vi "Main.vi"(10 "Acq Panel":refnum<vi>, 11 "Module Admin":refnum<class "Delacor_lib_QMH_Module Admin.lvclass">) -> ()   [LabVIEW 2019, in "Adquirir.lvlib"]
doc: "This template is based off of the Queued Message Handler design pattern and the Queued Message Handler project template that ships with LabVIEW.\n\nThe main difference is that the queue is private to this module and communication between modules is performed via Broadcast and Request events.\n\nRequest events are wrapped in public API methods and are handled in the Event Handling Loop (EHL) of this VI. Any module can register for Broadcast events sent by this module. The EHL generates messages based on user interface actions.\n\nThe Message Handling Loop (MHL) processes messages generated by the EHL, or by other messages. The messages are string values, so new messages can be added easily to the Message Cases case structure in the MHL. Each message cluster can also provide an optional value for Message Data, which is a variant that can be converted to whatever message-specific data is required.\n_____\nBased on Delacor QMH Project Template 5.0.0.82."
uses:
  Adquirir.lvlib
  <vilib>/Delacor/Delacor QMH/Libraries/Module Admin_class/Delacor_lib_QMH_Module Admin.lvclass
  Module Data--cluster.ctl
  Stop helper loop Argument--cluster.ctl
  <vilib>/Delacor/Delacor QMH/Libraries/Message Queue_class/Delacor_lib_QMH_Message Queue.lvclass/Delacor_lib_QMH_Message Queue.ctl
  Stop Argument--cluster.ctl
  <vilib>/Delacor/Delacor QMH/Libraries/Module Admin_class/Delacor_lib_QMH_Module Admin.lvclass/Delacor_lib_QMH_Module Admin.ctl
  <vilib>/Utility/miscctls.llb/LVPointTypeDef.ctl
  <vilib>/Delacor/Delacor QMH/Libraries/Message Queue_class/Delacor_lib_QMH_Enqueue Message (Single).vi
  <vilib>/Delacor/Delacor QMH/Libraries/Module Admin_class/Delacor_lib_QMH_Get External Launch.vi
  <vilib>/Utility/error.llb/Error Cluster From Error Code.vi
  <vilib>/ErrorRing/Error Ring.xnode
  <vilib>/Delacor/Delacor QMH/Libraries/Message Queue_class/Delacor_lib_QMH_Message Queue.lvclass
panel:
  out "Time Stamp":timestamp
  in  "Simulate MHL Error":bool
  in  "Simulate EHL Error":bool
  out "error out":errorcluster
  out "Status":string
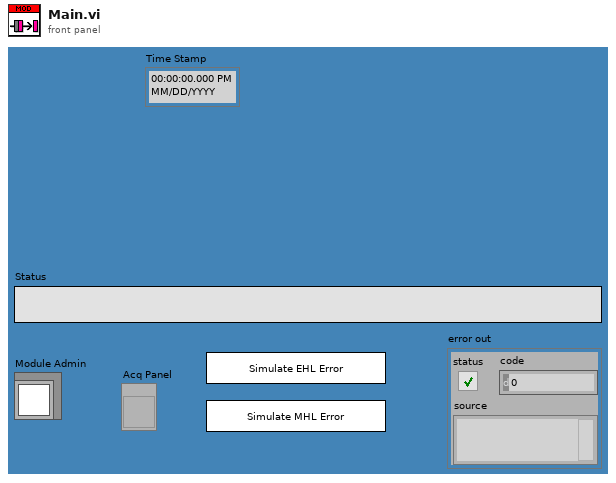
[diagram p1: front panel]
types:
  T1 = typedef "Adquirir.lvlib/Request Events--cluster.ctl" = cluster{"Stop Module":refnum<user-event>, "Show Panel":refnum<user-event>, "Hide Panel":refnum<user-event>, "Get Module Execution Status":refnum<user-event>, "Show Diagram":refnum<user-event>, "Start Helper Loop":refnum<user-event>, "Stop helper loop":refnum<user-event>}
  T2 = typedef "Adquirir.lvlib/Module Data--cluster.ctl" = cluster{"Status":string}
  T3 = typedef "Adquirir.lvlib/Stop helper loop Argument--cluster.ctl" = cluster{"Boolean":bool}
  T4 = enum32{"invalid lock state", "Not Locked", "Locked (No Password)", "Password-protected"}
  T5 = typedef "Adquirir.lvlib/Stop Argument--cluster.ctl" = cluster{"Origin":string, "Exit via Stop Module Req?":bool, "Wait for Module to stop?":bool}
  T6 = typedef "LVPointTypeDef.ctl" = cluster{"Horizontal":i16, "Vertical":i16}
  T7 = enum32{"Invalid", "Standard", "Closed", "Hidden", "Minimized", "Maximized"}
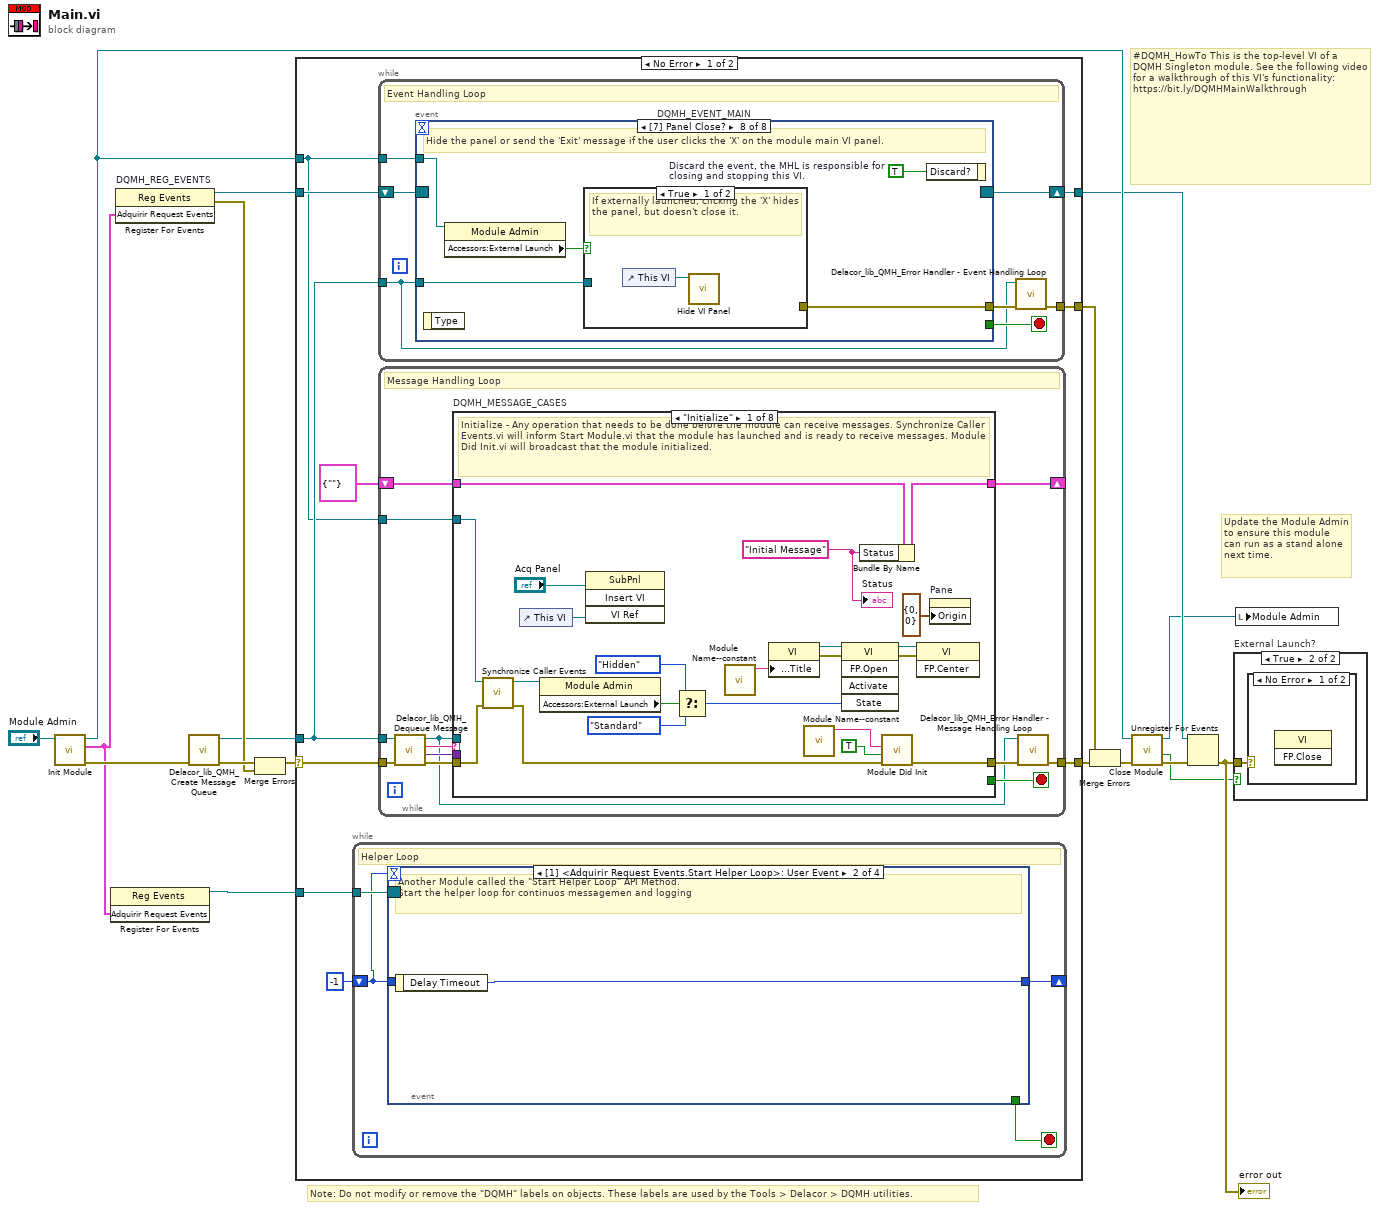
[diagram p0: block diagram]
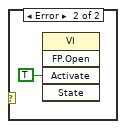
[diagram p3: hidden frame]
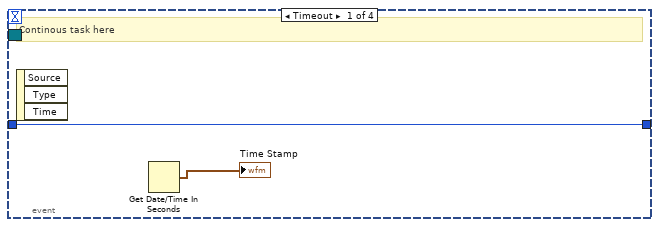
[diagram p4: hidden frame]
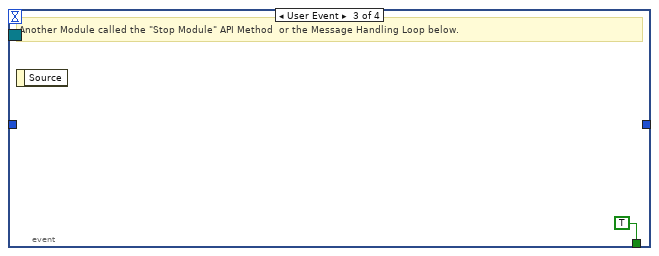
[diagram p5: hidden frame]
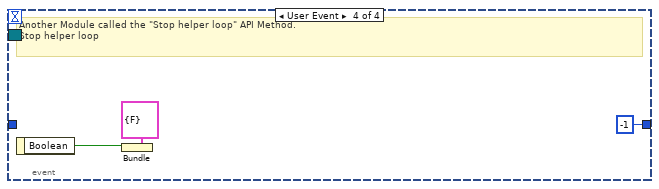
[diagram p6: hidden frame]
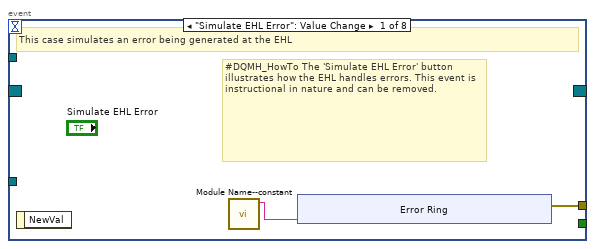
[diagram p7: hidden frame]
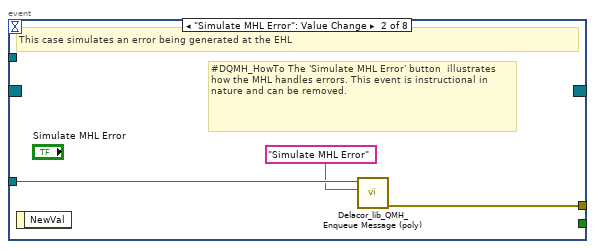
[diagram p8: hidden frame]
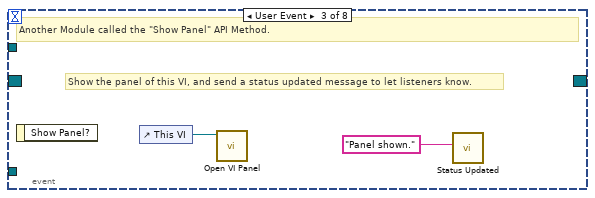
[diagram p9: hidden frame]
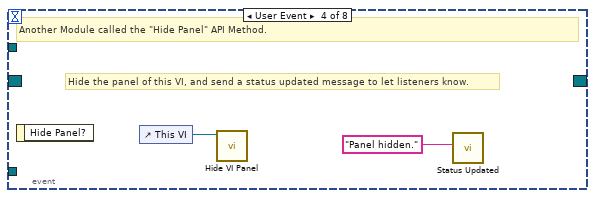
[diagram p10: hidden frame]
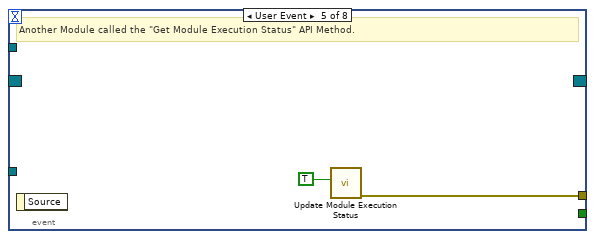
[diagram p11: hidden frame]
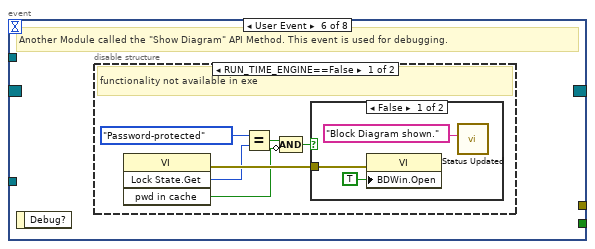
[diagram p12: hidden frame]
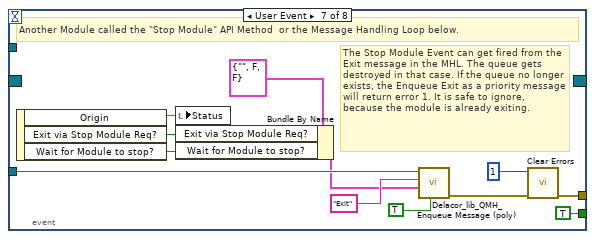
[diagram p15: hidden frame]
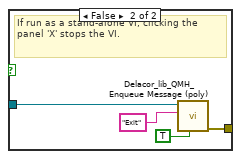
[diagram p16: hidden frame]
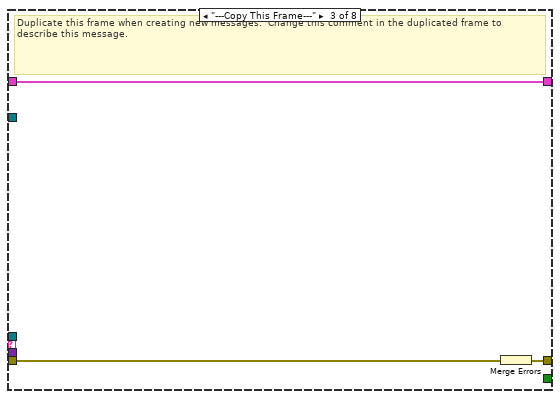
[diagram p18: hidden frame]
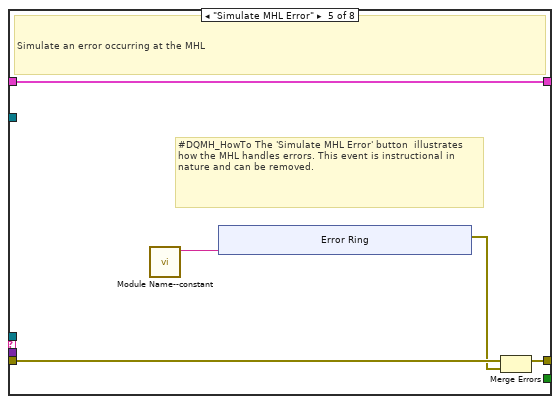
[diagram p20: hidden frame]
diagram:
  # "#DQMH_HowTo This is the top-level VI of a DQMH Singleton module. See the following video for a walkthrough of this VI's functionality: https://bit.ly/DQMHMainWalkthrough"
  # "Note: Do not modify or remove the \"DQMH\" labels on objects. These labels are used by the Tools > Delacor > DQMH utilities."
  # "Update the Module Admin to ensure this module can run as a stand alone next time."
  n1 = call "Init Module.vi"("Singleton Module Admin in"="Module Admin") -> ("error out"=w17:errorcluster, "Adquirir Request Events"=w1:T1, "Singleton Module Admin out"=w9:refnum<class "Delacor_lib_QMH_Module Admin.lvclass">)  [unwired: 8 in]
  n2 = register-events(w1) -> (reference out=w2:refnum<event-registration>)  [unwired: 2 in, 1 out]
  n3 = register-events "DQMH_REG_EVENTS"(w1) -> (reference out=w7:refnum<event-registration>, error out=w10:errorcluster)  [unwired: 2 in]
  n4 = call <vilib>:"Delacor_lib_QMH_Create Message Queue.vi"("error in (no error)"=w17) -> ("error out"=w12:errorcluster, "Message Queue"=w6:refnum<class "Delacor_lib_QMH_Message Queue.lvclass">)  [unwired: 9 in]
  n5 = Merge Errors(w12, w10) -> (w11:errorcluster)
  n6 = case shown="No Error" w11 {
    selector: w11 -> [w26 w197]
    tunnel: [w28 w196] -> w18
    tunnel: [w25 w202] -> w8
    tunnel: w7 -> [w23 w202]
    tunnel: w6 -> [w22 w195]
    tunnel: [w27 _] -> w15
    tunnel: w9 -> [w21 w198]
    tunnel: w2 -> [w20 _]
    frame No Error {
      n7 = while {
        tunnel: w20 -> [w32]
        shift-right: [w30] -> _
        shift-left: -1 -> [w29]
        stop <- w31 stop-if-true
        # "Helper Loop"
        n8 = event shown="[1] <Adquirir Request Events.Start Helper Loop>: User Event" {
          selector: w32 -> [_ _ _ _]
          dyn-events: _ -> [_ _ _ _]
          timeout: w29 -> [_ _ _ _]
          tunnel: [_ _ TRUE _] -> w31
          tunnel: [w34 w35 _ -1] -> w30
          tunnel: w29 -> [w34 _ _ _]
          event Timeout {
            # "Continous task here"
            n9 = event-data() -> ()  [unwired: 1 in, 3 out]
            n10 = Get Date/Time In Seconds() -> (seconds since 1Jan1904=→"Time Stamp":timestamp)
          }
          event User Event {
            # "Another Module called the \"Start Helper Loop\" API Method.\nStart the helper loop for continuos messagemen and logging"
            n11 = event-data() -> ("Delay Timeout"=w35:i32)  [unwired: 1 in]
          }
          event User Event {
            # "Another Module called the \"Stop Module\" API Method  or the Message Handling Loop below."
            n12 = event-data() -> ()  [unwired: 1 in, 1 out]
          }
          event User Event {
            # "Another Module called the \"Stop helper loop\" API Method.\nStop helper loop"
            n13 = event-data() -> ("Boolean"=w38:bool)  [unwired: 1 in]
            n14 = Bundle(cluster=T3 {"Boolean"=FALSE} ("Stop helper loop Argument"), "Boolean"=w38) -> ()  [unwired: 1 out]
          }
        }
      }
      n15 = while {
        tunnel: w22 -> [w40]
        shift-right: [w43] -> w25
        shift-left: w23 -> [w44]
        tunnel: [w45] -> w27
        tunnel: w21 -> [w41]
        stop <- w42 stop-if-true
        # "Event Handling Loop"
        n16 = event "DQMH_EVENT_MAIN" shown="[7] Panel Close?" {
          selector: w44 -> [_ _ _ _ _ _ _ _]
          dyn-events: [_ _ _ _ _ _ _ _] -> w43
          timeout: _ -> [_ _ _ _ _ _ _ _]
          tunnel: [_ _ _ _ _ _ TRUE ("Discard?") _] -> w42
          tunnel: w40 -> [_ w57 _ _ _ _ w81 w88]
          tunnel: [w48 w58 _ _ w64 _ w84 w90] -> w46
          tunnel: w41 -> [_ _ _ _ _ _ _ w87]
          event "Simulate EHL Error": Value Change {
            # "#DQMH_HowTo The 'Simulate EHL Error' button  illustrates how the EHL handles errors. This event is instructional in nature and can be removed."
            # "This case simulates an error being generated at the EHL"
            n17 = event-data() -> ()  [unwired: 1 in, 1 out]
            n18 = call "Module Name--constant.vi"() -> ("Module Name"=w47:string)  [unwired: 11 in]
            n19 = xnode "Error Ring"("parameter 0"=w47) -> ("error out"=w48:errorcluster)
          }
          event "Simulate MHL Error": Value Change {
            # "#DQMH_HowTo The 'Simulate MHL Error' button  illustrates how the MHL handles errors. This event is instructional in nature and can be removed."
            # "This case simulates an error being generated at the EHL"
            n20 = event-data() -> ()  [unwired: 1 in, 1 out]
            n21 = call-poly <vilib>:"Delacor_lib_QMH_Enqueue Message (poly).vi"("Message"="Simulate MHL Error", "Message Queue in"=w57) -> ("error out"=w58:errorcluster)  [unwired: 8 in, 1 out]
          }
          event User Event {
            # "Show the panel of this VI, and send a status updated message to let listeners know."
            # "Another Module called the \"Show Panel\" API Method."
            n22 = event-data() -> ()  [unwired: 1 in, 1 out]
            n23 = control-ref of="This VI"() -> (w60:refnum<vi>)
            n24 = call "Open VI Panel.vi"("VI"=w60) -> ()  [unwired: 10 in, 1 out]
            n25 = call "Status Updated.vi"("Status"="Panel shown." ("format string")) -> ()  [unwired: 10 in, 1 out]
          }
          event User Event {
            # "Hide the panel of this VI, and send a status updated message to let listeners know."
            # "Another Module called the \"Hide Panel\" API Method."
            n26 = event-data() -> ()  [unwired: 1 in, 1 out]
            n27 = control-ref of="This VI"() -> (w62:refnum<vi>)
            n28 = call "Hide VI Panel.vi"("VI"=w62) -> ()  [unwired: 10 in, 1 out]
            n29 = call "Status Updated.vi"("Status"="Panel hidden." ("format string")) -> ()  [unwired: 10 in, 1 out]
          }
          event User Event {
            # "Another Module called the \"Get Module Execution Status\" API Method."
            n30 = event-data() -> ()  [unwired: 1 in, 1 out]
            n31 = call "Update Module Execution Status.vi"("Running?"=TRUE) -> ("error out"=w64:errorcluster)  [unwired: 10 in]
          }
          event User Event {
            # "Another Module called the \"Show Diagram\" API Method. This event is used for debugging."
            n32 = event-data() -> ()  [unwired: 1 in, 1 out]
            n33 = disable-structure shown="RUN_TIME_ENGINE==False" {
              frame condition #0 (active) {
                # "functionality not available in exe"
                n34 = invoke class="VI" method="Lock State.Get"() -> (error out=w70:errorcluster, "Get Lock State"=w69:T4, "pwd in cache"=w66:bool)  [unwired: 4 in, 1 out]
                n35 = Equal?(x=T4."Password-protected", y=w69) -> (x = y?=w67:bool)
                n36 = Compound Arithmetic op=AND(w67, invert w66) -> (w65:bool)
                n37 = case shown="False" w65 {
                  tunnel: w70 -> [w73 _]
                  frame False {
                    n38 = property class="VI"(error in=w73, "BDWin.Open"=TRUE ("Block Diagram Window:Open")) -> ()  [unwired: 1 in, 2 out]
                    n39 = call "Status Updated.vi"("Status"="Block Diagram shown." ("format string")) -> ()  [unwired: 10 in, 1 out]
                  }
                  frame True {
                    # "Password-protected VI, and the password is not in the cache. Do not show the diagram."
                  }
                }
              }
              frame condition #1 {
              }
            }
          }
          event User Event {
            # "The Stop Module Event can get fired from the Exit message in the MHL. The queue gets destroyed in that case. If the queue no longer exists, the Enqueue Exit as a priority message will return error 1. It is safe to ignore, because the module is already exiting."
            # "Another Module called the \"Stop Module\" API Method  or the Message Handling Loop below."
            n40 = event-data() -> ("Origin"=w80:string, "Exit via Stop Module Req?"=w76:bool, "Wait for Module to stop?"=w75:bool)  [unwired: 1 in]
            n41 = local write "Status"(w80) -> ()
            n42 = Bundle By Name(cluster=T5 {"Origin"="", "Exit via Stop Module Req?"=FALSE, "Wait for Module to stop?"=FALSE} ("Stop Argument"), "Exit via Stop Module Req?"=w76, "Wait for Module to stop?"=w75) -> (w74:T5)
            n43 = call-poly <vilib>:"Delacor_lib_QMH_Enqueue Message (poly).vi"("Priority Message? (F)"=TRUE, "Message Data"=w74, "Message"="Exit", "Message Queue in"=w81) -> ("error out"=w85:errorcluster)  [unwired: 6 in, 1 out]
            n44 = call <vilib>:"Clear Errors.vi"("error in (no error)"=w85, "specific error code to clear (0: all)"=1) -> ("error out"=w84:errorcluster)  [unwired: 4 in, 1 out]
          }
          event Panel Close? {
            w89 = TRUE  # Discard the event, the MHL is responsible for closing and stopping this VI.
            # "Hide the panel or send the 'Exit' message if the user clicks the 'X' on the module main VI panel."
            n45 = event-data() -> ()  [unwired: 1 in, 1 out]
            n46 = property class="Module Admin"(reference=w87) -> ("Accessors:External Launch"=w86:bool)  [unwired: 1 in, 2 out]
            n47 = case shown="True" w86 {
              tunnel: w88 -> [_ w94]
              tunnel: [_ w95] -> w90
              frame True {
                # "If externally launched, clicking the 'X' hides the panel, but doesn't close it."
                n48 = control-ref of="This VI"() -> (w91:refnum<vi>)
                n49 = call "Hide VI Panel.vi"("VI"=w91) -> ()  [unwired: 10 in, 1 out]
              }
              frame False {
                # "If run as a stand-alone VI, clicking the panel 'X' stops the VI."
                n50 = call-poly <vilib>:"Delacor_lib_QMH_Enqueue Message (poly).vi"("Priority Message? (F)"=TRUE, "Message"="Exit", "Message Queue in"=w94) -> ("error out"=w95:errorcluster)  [unwired: 7 in, 1 out]
              }
            }
            n51 = event-data("Discard?"=w89) -> ()  [unwired: 1 in, 1 out]
          }
        }
        n52 = call-dynamic "Delacor_lib_QMH_Error Handler - Event Handling Loop.vi"("error in (no error)"=w46, "Message Queue in"=w40) -> ("dup error in"=w45:errorcluster)  [unwired: 8 in, 1 out]
      }
      n53 = while {
        tunnel: w22 -> [w98]
        shift-right: [w102] -> _
        shift-left: T2 {"Status"=""} ("Data Cluster") -> [w103]
        tunnel: w26 -> [w106]
        tunnel: [w104] -> w28
        tunnel: w21 -> [w96]
        stop <- w101 stop-if-true
        # "Message Handling Loop"
        n54 = call-dynamic "Delacor_lib_QMH_Dequeue Message.vi"("error in (no error)"=w106, "Message Queue in"=w98) -> ("error out"=w105:errorcluster, "Message Data"=w99:variant, "Message"=w100:string, "Message Queue out"=w97:refnum<class "Delacor_lib_QMH_Message Queue.lvclass">)  [unwired: 6 in]
        n55 = case "DQMH_MESSAGE_CASES" shown="\"Initialize\"" w100 {
          selector: w100 -> [_ _ _ _ _ _ _ w182]
          tunnel: w97 -> [_ _ _ _ _ w152 w174 _]
          tunnel: w105 -> [w127 w131 w134 w136 w141 w159 w180 w184]
          tunnel: [w125 w131 w133 w136 w140 w155 w177 w185] -> w107
          tunnel: w103 -> [w116 w130 w132 w135 w138 w154 w173 w183]
          tunnel: [w115 w130 w132 w135 w138 w154 w173 w183] -> w102
          tunnel: [_ _ _ _ _ _ w172 _] -> w101
          tunnel: w99 -> [_ _ _ _ _ w153 w171 _]
          tunnel: w96 -> [w117 _ _ _ _ w151 w166 _]
          frame "Initialize" {
            w110 = "Initial Message" ("Initial Message")
            # "Initialize - Any operation that needs to be done before the module can receive messages. Synchronize Caller Events.vi will inform Start Module.vi that the module has launched and is ready to receive messages. Module Did Init.vi will broadcast that the module initialized."
            n56 = call "Synchronize Caller Events.vi"("error in (no error)"=w127, "Singleton Module Admin in"=w117) -> ("error out"=w126:errorcluster, "Singleton Module Admin out"=w112:refnum<class "Delacor_lib_QMH_Module Admin.lvclass">)  [unwired: 8 in]
            n57 = control-ref of="This VI"() -> (w108:refnum<vi>)
            n58 = property class="Module Admin"(reference=w112) -> ("Accessors:External Launch"=w121:bool)  [unwired: 1 in, 2 out]
            n59 = invoke class="SubPnl" method="Insert VI"(reference="Acq Panel", "VI Ref"=w108) -> ()  [unwired: 2 in, 4 out]
            n60 = Select(t=T7."Hidden" ("State"), s=w121, f=T7."Standard" ("State")) -> (s? t:f=w118:T7)
            n61 = call "Module Name--constant.vi"() -> ("Module Name"=w124:string)  [unwired: 11 in]
            n62 = property class="VI"("Front Panel.Title"=w124) -> (reference out=w123:refnum<vi>, error out=w129:errorcluster)  [unwired: 2 in]
            n63 = call "Module Name--constant.vi"() -> ("Module Name"=w113:string)  [unwired: 11 in]
            n64 = invoke class="VI" method="FP.Open"(reference=w123, error in=w129, "State"=w118) -> (reference out=w122:refnum<vi>, error out=w128:errorcluster)  [unwired: 2 in, 3 out]
            n65 = Bundle By Name(cluster=w116, "Status"=w110) -> (w115:T2)
            n66 = call "Module Did Init.vi"("error in (no error)"=w126, "Initialized?"=TRUE, "Origin"=w113) -> ("error out"=w125:errorcluster)  [unwired: 8 in]
            n67 = invoke class="VI" method="FP.Center"(reference=w122, error in=w128) -> ()  [unwired: 1 in, 3 out]
            n68 = property on="Pane" class="Pane"("Origin"=T6 {"Horizontal"=0, "Vertical"=0}) -> ()  [unwired: 2 in, 2 out]
            "Status" <- w110
          }
          frame "--- Module Specific ---" {
            # "Separator -- The following cases handle messages specific to this Module."
          }
          frame "---Copy This Frame---" {
            # "Duplicate this frame when creating new messages.  Change this comment in the duplicated frame to describe this message."
            n69 = Merge Errors(w134) -> (w133:errorcluster)
          }
          frame "--- Exit and Error Handling---" {
            # "Separator - The following cases handle errors and exit messages."
          }
          frame "Simulate MHL Error" {
            # "#DQMH_HowTo The 'Simulate MHL Error' button  illustrates how the MHL handles errors. This event is instructional in nature and can be removed."
            # "Simulate an error occurring at the MHL"
            n70 = call "Module Name--constant.vi"() -> ("Module Name"=w137:string)  [unwired: 11 in]
            n71 = xnode "Error Ring"("parameter 0"=w137) -> ("error out"=w139:errorcluster)
            n72 = Merge Errors(w141, w139) -> (w140:errorcluster)
          }
          frame "Error" {
            # "#CodeRecommended - If you ever change the name of this \"Error\" message, you'll need to update the name in the Check Loop Error.vi as well."
            # "#CodeRecommended - If the module is running in standalone mode (External Launch = FALSE), this code will pop up an error dialog and call the 'Exit' message if an error occurs. Add more fine-grained error handling here."
            # "Error - Check the error message data and respond accordingly. This message is sent by the \"Error Handler\" VIs at the end of each loop in this application."
            n73 = property class="Module Admin"(reference=w151) -> ("Accessors:External Launch"=w150:bool)  [unwired: 1 in, 2 out]
            n74 = Variant To Data(error in=w159, type=errorcluster {"status"=FALSE, "code"=0, "source"=""} ("error constant"), Variant=w153) -> (data=w160:errorcluster, error out=w157:errorcluster)
            n75 = call "Module Name--constant.vi"() -> ("Module Name"=w149:string)  [unwired: 11 in]
            n76 = call "Error Reported.vi"("Additional Information"=w149, "Error"=w160) -> ()  [unwired: 9 in, 1 out]
            n77 = case shown="False" w150 {
              tunnel: [w165 _] -> w156
              tunnel: w152 -> [w163 _]
              tunnel: w160 -> [w164 _]
              frame False {
                # "If the module is running standalone, then pop up an error dialog and call the \"Exit\" message."
                n78 = call <vilib>:"Simple Error Handler.vi"("error in (no error)"=w164) -> ()  [unwired: 4 in, 5 out]
                n79 = call-poly <vilib>:"Delacor_lib_QMH_Enqueue Message (poly).vi"("Priority Message? (F)"=TRUE, "Message"="Exit", "Message Queue in"=w163) -> ("error out"=w165:errorcluster)  [unwired: 7 in, 1 out]
              }
              frame True {
                # "If the module was launched externally, calling the Error Reported broadcast VI is the only action performed by the \"Error\" message. The module's caller can then process the error appropriately."
              }
            }
            n80 = Merge Errors(w157, w156) -> (w155:errorcluster)
            n81 = local write "error out"(w155) -> ()
          }
          frame "Exit" {
            w170 = 91  # 91: not all Exit messages will have an argument
            w172 = TRUE  # Stop the VI
            # "Release the message queue reference"
            # "#CodeNeeded - Add any required cleanup code here"
            # "Exit - Exit the application."
            n82 = Variant To Data(error in=w180, type=T5 {"Origin"="", "Exit via Stop Module Req?"=FALSE, "Wait for Module to stop?"=FALSE} ("Stop Argument"), Variant=w171) -> (data=w168:T5, error out=w176:errorcluster)
            n83 = call <vilib>:"Clear Errors.vi"("error in (no error)"=w176, "specific error code to clear (0: all)"=w170) -> ("error out"=w179:errorcluster)  [unwired: 4 in, 1 out]
            n84 = control-ref of="This VI"() -> (w167:refnum<vi>)
            n85 = call-dynamic "Delacor_lib_QMH_Release Message Queue.vi"("error in (no error)"=w179, "Message Queue"=w174) -> ("error out"=w178:errorcluster)  [unwired: 9 in]
            n86 = call "Handle Exit.vi"("Stop Argument"=w168, "Admin in"=w166, "VI reference"=w167) -> ("error out"=w175:errorcluster)  [unwired: 7 in, 1 out]
            n87 = Merge Errors(w178, w175) -> (w177:errorcluster)
          }
          frame Default {
            # "'Default' case only runs if there is a message that isn't defined in any of the other cases.  Output a programming error."
            n88 = call "Module Name--constant.vi"() -> ("Module Name"=w181:string)  [unwired: 11 in]
            n89 = xnode "Error Ring"("parameter 0"=w182, "parameter 1"=w181) -> ("error out"=w186:errorcluster)
            n90 = Merge Errors(w184, w186) -> (w185:errorcluster)
          }
        }
        n91 = call-dynamic "Delacor_lib_QMH_Error Handler - Message Handling Loop.vi"("error in (no error)"=w107, "Message Queue in"=w97) -> ("dup error in"=w104:errorcluster)  [unwired: 8 in, 1 out]
      }
    }
    frame Error {
      # "Synchronize Caller Events.vi will inform Start Module.vi that the module has launched and will let the code calling Start Module.vi register for broadcasts and would permit the caller receive the broadcast that an error occurred at launch time."
      n92 = call-dynamic "Delacor_lib_QMH_Release Message Queue.vi"("error in (no error)"=w197, "Message Queue"=w195) -> ("error out"=w196:errorcluster)  [unwired: 9 in]
      n93 = call "Synchronize Caller Events.vi"("Singleton Module Admin in"=w198) -> ("error out"=w203:errorcluster)  [unwired: 9 in, 1 out]
      n94 = call "Module Name--constant.vi"() -> ("Module Name"=w201:string)  [unwired: 11 in]
      n95 = Format Into String(format string="An error occurred during initialization. %s is no longer running.", w201) -> (resulting string=w199:string)  [unwired: 2 in, 1 out]
      n96 = Merge Errors(w196, w203) -> (w204:errorcluster)
      n97 = call "Error Reported.vi"("Additional Information"=w199, "Error"=w204) -> ()  [unwired: 9 in, 1 out]
    }
  }
  n98 = Merge Errors(w15, w18) -> (w14:errorcluster)
  n99 = call "Close Module.vi"("error in (no error)"=w14, "Module Admin in"=w9) -> ("error out"=w16:errorcluster, "External Launch"=w3:bool, "Module Admin out"=w4:refnum<class "Delacor_lib_QMH_Module Admin.lvclass">)  [unwired: 7 in]
  n100 = Unregister For Events(event registration refnum=w8, error in=w16) -> (error out=w13:errorcluster)
  "error out" <- w13
  n101 = case "External Launch?" shown="True" w3 {
    tunnel: w13 -> [_ w205]
    frame False {
    }
    frame True {
      n102 = case shown="No Error" w205 {
        frame No Error {
          n103 = invoke class="VI" method="FP.Close"() -> ()  [unwired: 3 in, 3 out]
        }
        frame Error {
          n104 = invoke class="VI" method="FP.Open"("Activate"=TRUE ("Activate?")) -> ()  [unwired: 4 in, 5 out]
        }
      }
    }
  }
  n105 = local write "Module Admin"(w4) -> ()
